vi "Topic_Gripper.vi"(11 "Side":T1) -> (3 "Definitions":T2={"Topic"="", "Type"="", "Action"=enum."Node", "Update (ms)"=1, "write queue"=1})   [LabVIEW 2010]
uses:
  <userlib>/ROSforLV/ROS/Code/Console/Servers/ServerSubs/TopicDef.ctl
  <userlib>/ROSforLV/ROS/Code/SubVIs/_ROSDirection.ctl
  <userlib>/ROSforLV/ROS/Code/SubVIs/BaxterSide.ctl
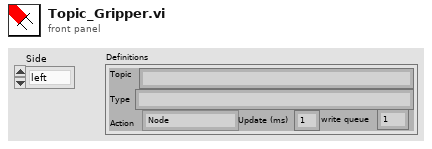
[diagram p1: front panel]
types:
  T1 = typedef "BaxterSide.ctl" = enum16{"left", "right"}
  T2 = typedef "TopicDef.ctl" = cluster{"Topic":string, "Type":string, "Action":T3, "Update (ms)":u16, "write queue":u16}
  T3 = typedef "_ROSDirection.ctl" = enum16{"Node", "Publisher", "Subscriber", "Service Client"}
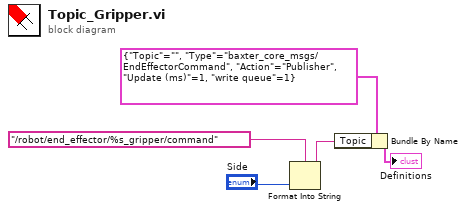
[diagram p0: block diagram]
diagram:
  n1 = Format Into String(format string="/robot/end_effector/%s_gripper/command" ("Topic"), "Side") -> (resulting string=w3:string)  [unwired: 2 in, 1 out]
  n2 = Bundle By Name(cluster=T2 {"Topic"="", "Type"="baxter_core_msgs/EndEffectorCommand", "Action"=enum."Publisher", "Update (ms)"=1, "write queue"=1} ("Definitions"), "Topic"=w3) -> (→"Definitions":T2)
